vi "DeadZone.vi"(1 "Multiplier":dbl=1.0, 2 "DeadZone":dbl, 3 "Points(in)":cluster{"X":dbl, "Y":dbl}) -> (0 "Points(out)":cluster{"X":dbl, "Y":dbl})   [LabVIEW 2012]
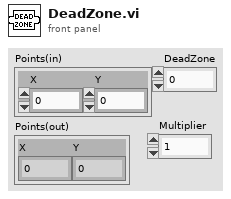
[diagram p1: front panel]
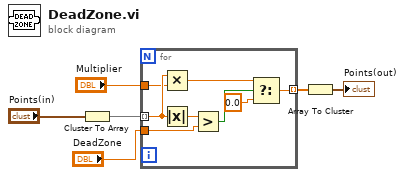
[diagram p0: block diagram]
diagram:
  n1 = Cluster To Array(cluster="Points(in)") -> (array=w5:dbl[])
  n2 = for {
    tunnel: w5 -> [w10] mode=indexing
    tunnel: [w9] -> w4 mode=indexing
    tunnel: "DeadZone" -> [w13]
    tunnel: "Multiplier" -> [w7]
    n3 = Multiply(x=w10, y=w7) -> (x*y=w8:dbl)
    n4 = Absolute Value(x=w10) -> (abs(x)=w14:dbl)
    n5 = Greater?(x=w14, y=w13) -> (0:w12:bool)
    n6 = Select(t=w8, s=w12, f=0.0) -> (s? t:f=w9:dbl)
  }
  n7 = Array To Cluster(array=w4) -> (cluster=→"Points(out)":cluster{"[0]":dbl, "[1]":dbl})
